vi "PicoScope5000aExampleBlock.vi"() -> ()   [LabVIEW 2016]
panel:
  in  "Acquisition Settings":T1={"preTriggerSamples"=0, "postTriggerSamples"=1000, "timebase"=2, "Down-Sample Mode"=0, "Down Sample Ratio"=1} {"Down Sample Ratio" min=1 step=1; "Down-Sample Mode" items=["None"=0, "Aggregate"=1, "Decimate"=2, "Average"=4]}
  in  "Serial Number":string
  in  "Open using Serial Number":bool
  out "Channel B":i16[](graph)
  in  "Channel B Settings":T2={"Enabled"=FALSE, "Coupling"=1, "Range"=6, "Analogue Offset"=0.0} {"Range" items=["10 mV", "20 mV", "50 mV", "100 mV", "200 mV", "500 mV", "1 V", "2 V", "5 V", "10 V", "20 V", "50 V ", "100 V"]; "Coupling" items=["AC", "DC"]}
  in  "Resolution":i32(ring) items=["8-bit", "12-bit", "14-bit", "15-bit (max. 2 ch.)", "16-bit (max. 1 ch.)"]
  in  "PS5X4XA/B devices \nUSB Powered":bool=TRUE
  in  "Trigger Settings":T3={"Trigger Enabled"=TRUE, "Trigger Source"=enum."Channel A", "Trigger Threshold (16-bit counts)"=16384, "Trigger Direction"=2, "Trigger Delay (samples)"=0, "Auto Trigger Time (ms)"=0} {"Trigger Direction" items=["Rising"=2, "Falling"=3]}
  in  "Channel A Settings":T2={"Enabled"=TRUE, "Coupling"=1, "Range"=6, "Analogue Offset"=0.0} {"Range" items=["10 mV", "20 mV", "50 mV", "100 mV", "200 mV", "500 mV", "1 V", "2 V", "5 V", "10 V", "20 V", "50 V ", "100 V"]; "Coupling" items=["AC", "DC"]}
  in  "stop":bool
  out "Channel A":i16[](graph)
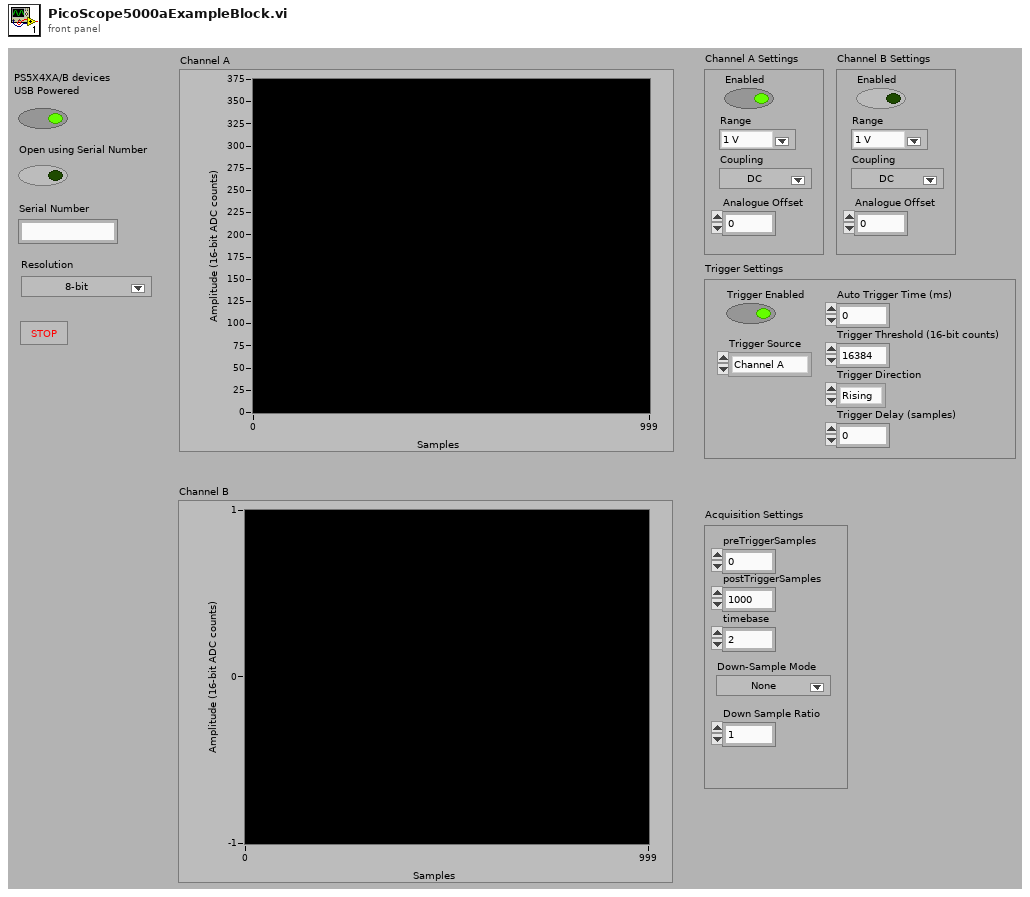
[diagram p1: front panel]
types:
  T1 = cluster{"preTriggerSamples":i32, "postTriggerSamples":i32, "timebase":u32, "Down-Sample Mode":u32, "Down Sample Ratio":u32}
  T2 = cluster{"Enabled":bool, "Coupling":i16, "Range":u16, "Analogue Offset":sgl}
  T3 = cluster{"Trigger Enabled":bool, "Trigger Source":enum16{"Channel A", "Channel B", "Channel C", "Channel D", "Ext."}, "Trigger Threshold (16-bit counts)":i16, "Trigger Direction":u16, "Trigger Delay (samples)":u32, "Auto Trigger Time (ms)":i16}
  T4 = cluster{"Channel D Buffer":i16[], "Channel C Buffer":i16[], "Channel B Buffer":i16[], "Channel A Buffer":i16[]}
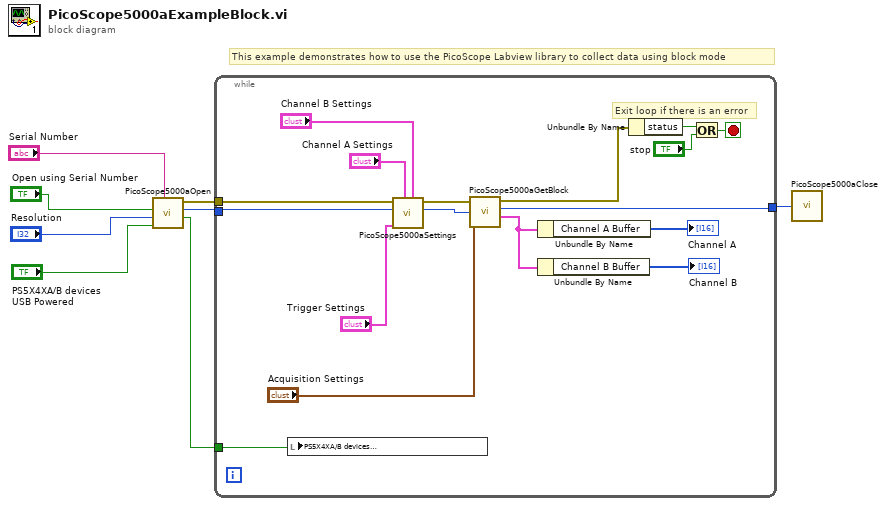
[diagram p0: block diagram]
diagram:
  # "This example demonstrates how to use the PicoScope Labview library to collect data using block mode"
  n1 = call "PicoScope5000aOpen.vi"("Serial Number"="Serial Number", "USB Powered Selection"="PS5X4XA/B devices \nUSB Powered", "Resolution"="Resolution", "Use Serial Number"="Open using Serial Number") -> ("USB Powered Indication"=w5:bool, "handle"=w6:i16, "error out"=w7:errorcluster)  [unwired: 3 in, 2 out]
  n2 = while {
    tunnel: w6 -> [w22]
    tunnel: w7 -> [w21]
    tunnel: [w20] -> w8
    tunnel: w5 -> [w13]
    stop <- w25 stop-if-true
    # "Exit loop if there is an error"
    n3 = local write "PS5X4XA/B devices \nUSB Powered"(w13) -> ()
    n4 = call "PicoScope5000aSettings.vi"("Channel B Settings"="Channel B Settings", "Channel A Settings"="Channel A Settings", "Trigger Settings"="Trigger Settings", "handle in"=w22, "error in"=w21) -> ("handle out"=w18:i16, "error out"=w17:errorcluster)  [unwired: 5 in]
    n5 = call "PicoScope5000aGetBlock.vi"("error in"=w17, "handle in"=w18, "Acquisition Settings"="Acquisition Settings") -> ("error out"=w19:errorcluster, "handle out"=w20:i16, "Buffers (Max or non-aggregated)"=w11:T4)  [unwired: 2 in, 3 out]
    n6 = Unbundle By Name(w11) -> ("Channel A Buffer"=→"Channel A":i16[])
    n7 = Unbundle By Name(w11) -> ("Channel B Buffer"=→"Channel B":i16[])
    n8 = Unbundle By Name(w19) -> ("status"=w16:bool)
    n9 = Or(x=w16, y="stop") -> (x .or. y?=w25:bool)
  }
  n10 = call "PicoScope5000aClose.vi"("handle"=w8) -> ()
